vi "locate tag by name.vi"(8 "error in":errorcluster, 10 "tag name":string, 11 "engine configuration in":refnum<class "engine configuration.lvclass">) -> (0 "error out":errorcluster, 2 "tag descriptor":refnum<class "tag descriptor.lvclass">, 3 "engine configuration out":refnum<class "engine configuration.lvclass">)   [LabVIEW 2013, in "engine configuration.lvclass"]
uses:
  engine configuration.lvclass
  <vilib>/NI/Tag Bus/tag/tag descriptor.lvclass
  engine configuration.lvclass/engine configuration.ctl
  <vilib>/NI/Tag Bus/tag/tag descriptor.lvclass/tag descriptor.ctl
  <vilib>/NI/Tag Bus/tag/read tag name.vi
  <vilib>/NI/CEF/CEF_TreeControl/NISE_CEF_TreeControl.lvlib
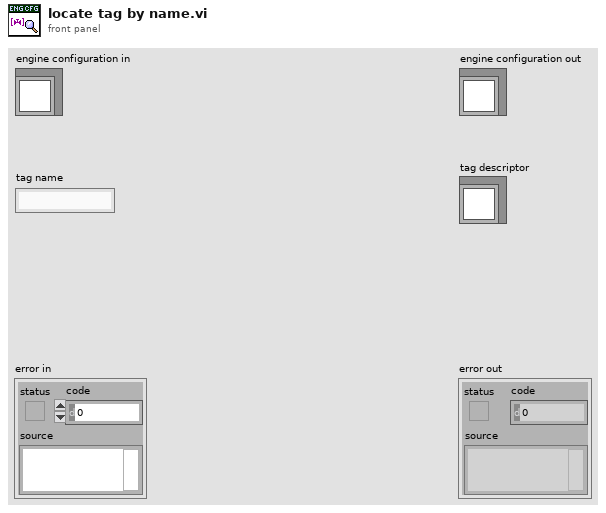
[diagram p1: front panel]
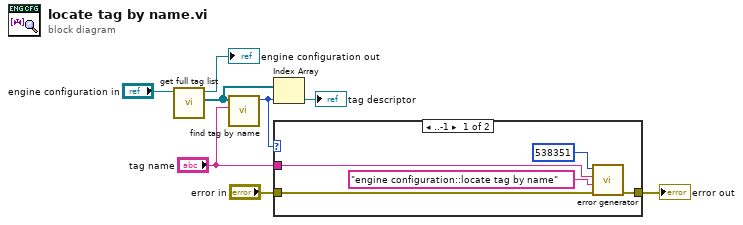
[diagram p0: block diagram]
diagram:
  n1 = call "get full tag list.vi"("engine configuration in"="engine configuration in") -> ("tag list"=w3:refnum<class "tag descriptor.lvclass">[], "engine configuration out"=→"engine configuration out":refnum<class "engine configuration.lvclass">)  [unwired: 9 in]
  n2 = call <vilib>:"find tag by name.vi"("name"="tag name", "tags in"=w3) -> ("index"=w2:i32)  [unwired: 9 in]
  n3 = Index Array(array=w3, index=w2) -> (element=→"tag descriptor":refnum<class "tag descriptor.lvclass">)
  n4 = case shown="..-1" w2 {
    tunnel: "error in" -> [w12 w14]
    tunnel: [w13 w14] -> w5
    tunnel: "tag name" -> [w10 _]
    frame ..-1 {
      n5 = call <vilib>:"error generator.vi"("error in"=w12, "source"="engine configuration::locate tag by name", "append error message"=w10, "error code (0)"=538351) -> ("error out"=w13:errorcluster)  [unwired: 5 in]
    }
    frame 0.. {
    }
  }
  "error out" <- w5
